vi "RT Main.vi"() -> ()   [LabVIEW 2021]
uses:
  <vilib>/FPGAPlugInAG/myRIO-1900/niLvFpga_Open_myRIO-1900.vi
  <vilib>/rvi/interface/common/dynamic/niFpgaDynamicAddResources.vi
  <vilib>/rvi/interface/common/niFpgaWaitOnOcc.vi
  <vilib>/Utility/error.llb/Error Cluster From Error Code.vi
  <vilib>/rvi/errors/niLvFpgaAdjustHostInterfaceError.vi
  <vilib>/FPGAPlugInAG/Dynamic/niLvFpga_Close_Dynamic.vi
  <vilib>/rvi/interface/nirviOpenFPGA/nirviOpenFPGA.xnode
  FPGA Bitfiles/dmafifoproject_FPGATarget_FPGA_+Bf8FZcda64.lvbitx
  <vilib>/rvi/interface/nirviMethod/nirviMethod.xnode
  <vilib>/rvi/interface/nirviReadWriteControl/nirviReadWriteControl.xnode
  <vilib>/rvi/interface/nirviCloseFPGA/nirviCloseFPGA.xnode
  <vilib>/rvi/errors/niLvFpgaMergeErrorWithErrorCode.vi
  <vilib>/FPGAPlugInAG/Dynamic/niLvFpga_ConfigureFifo_Dynamic.vi
  NiFpgaLv.dll
  <vilib>/rvi/interface/Simulation/niFpgaSimulationCallBeginRW.vi
  <vilib>/FPGAPlugInAG/Dynamic/niLvFpga_ReadFifo_Dynamic.vi
  <vilib>/FPGAPlugInAG/Dynamic/niLvFpga_WriteFifo_Dynamic.vi
panel:
  out "Waveform Chart":i16[][](graph)
  in  "min loop time [ms]":u32
  in  "stop":bool
  out "measured loop time [ms]":u32
  in  "gain":sgl
  out "to RT-Elements Remaining":u32
  in  "audio frame size [sample]":u32
  out "From RT underflow?":bool
  out "to RT overflow":bool
  out "audio sampling interval [us]":u32
  in  "audio sampling rate":dbl
  out "from RT-depth":u32
  out "to RT-depth":u32
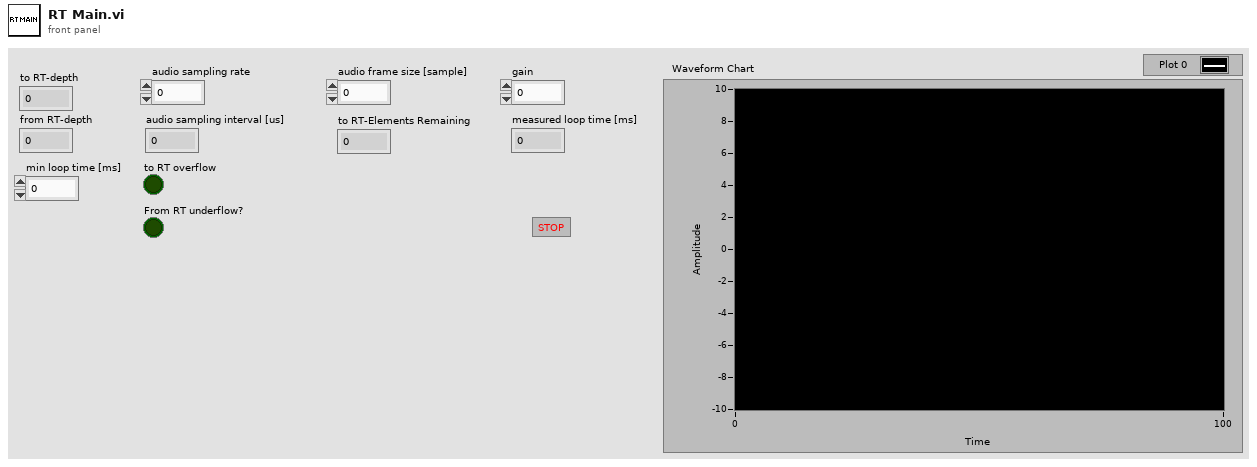
[diagram p1: front panel]
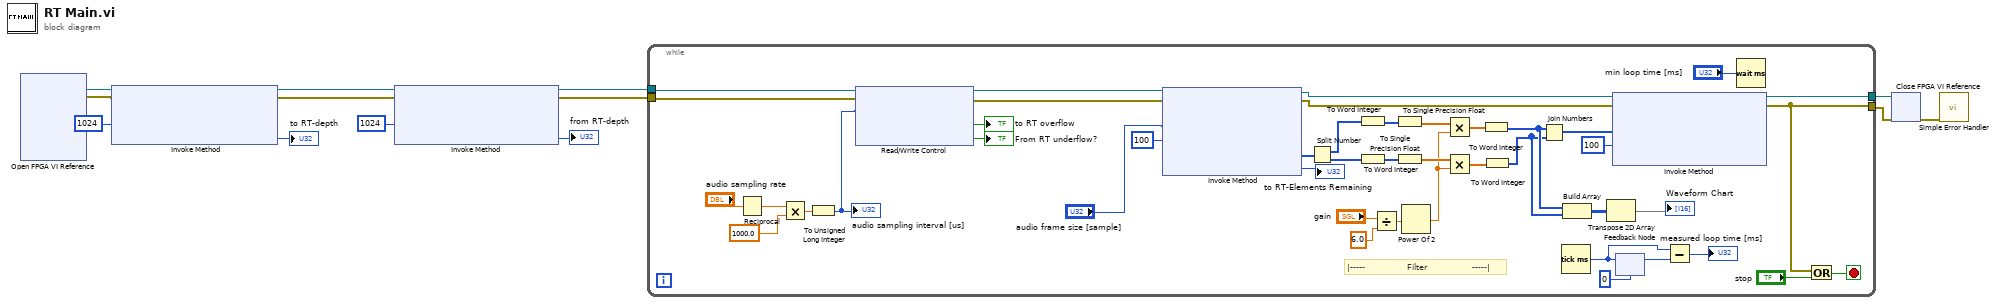
[diagram p0: block diagram]
diagram:
  n1 = xnode "Open FPGA VI Reference"() -> ("FPGA VI Reference Out"=w13:refnum<k20>, "error out"=w10:errorcluster)  [unwired: 2 in]
  n2 = xnode "Invoke Method"("FPGA VI Reference In"=w13, "error in"=w10, "Requested Depth"=u32 1024) -> ("FPGA VI Reference Out"=w12:refnum<k20>, "error out"=w11:errorcluster, "Actual Depth"=→"to RT-depth":u32)
  n3 = xnode "Invoke Method"("FPGA VI Reference In"=w12, "error in"=w11, "Requested Depth"=u32 1024) -> ("FPGA VI Reference Out"=w5:refnum<k20>, "error out"=w4:errorcluster, "Actual Depth"=→"from RT-depth":u32)
  n4 = while {
    tunnel: w5 -> [w57]
    tunnel: w4 -> [w56]
    tunnel: [w16] -> w3
    tunnel: [w17] -> w2
    stop <- w18 stop-if-true
    # "|-----              Filter               -----|"
    n5 = Reciprocal(x="audio sampling rate") -> (1/x=w52:dbl)
    n6 = Multiply(x=w52, y=1000.0) -> (x*y=w50:dbl)
    n7 = To Unsigned Long Integer(number=w50) -> (unsigned 32bit integer=w49:u32)
    "audio sampling interval [us]" <- w49
    n8 = xnode "Read/Write Control"("FPGA VI Reference In"=w57, "error in"=w56, "loop time(uSec)"=w49) -> ("FPGA VI Reference Out"=w55:refnum<k20>, "error out"=w54:errorcluster, "to RT overflow"=→"to RT overflow":bool, "From RT underflow?"=→"From RT underflow?":bool)
    n9 = xnode "Invoke Method"("FPGA VI Reference In"=w55, "error in"=w54, "Number of Elements"="audio frame size [sample]", "Timeout (ms)"=100) -> ("FPGA VI Reference Out"=w30:refnum<k20>, "error out"=w29:errorcluster, "Data"=w44:u32[], "Elements Remaining"=→"to RT-Elements Remaining":u32)
    n10 = Split Number(x=w44) -> (hi(x)=w42:u16[], lo(x)=w41:u16[])
    n11 = To Word Integer(number=w42) -> (16bit integer=w40:i16[])
    n12 = To Word Integer(number=w41) -> (16bit integer=w39:i16[])
    n13 = Divide(x="gain", y=sgl 6.0) -> (x/y=w34:sgl)
    n14 = To Single Precision Float(number=w40) -> (single precision float=w38:sgl[])
    n15 = To Single Precision Float(number=w39) -> (single precision float=w37:sgl[])
    n16 = Power Of 2(x=w34) -> (2^x=w33:sgl)
    n17 = Multiply(x=w38, y=w33) -> (x*y=w32:sgl[])
    n18 = Multiply(x=w37, y=w33) -> (x*y=w31:sgl[])
    n19 = To Word Integer(number=w32) -> (16bit integer=w26:i16[])
    n20 = To Word Integer(number=w31) -> (16bit integer=w25:i16[])
    n21 = Join Numbers(hi=w26, lo=w25) -> ((hi.lo)=w28:u32[])
    n22 = Tick Count (ms)() -> (millisecond timer value=w21:u32)
    n23 = Build Array(w26, w25) -> (w24:i16[][])
    n24 = Transpose 2D Array(2D array=w24) -> (transposed array=→"Waveform Chart":i16[][])
    n25 = xnode "Invoke Method"("FPGA VI Reference In"=w30, "error in"=w29, "Data"=w28, "Timeout (ms)"=100) -> ("FPGA VI Reference Out"=w16:refnum<k20>, "error out"=w17:errorcluster)  [unwired: 1 out]
    n26 = feedback-in #1(w21) -> ()
    n27 = feedback #1(u32 0 ("millisecond timer value")) -> (w22:u32)
    n28 = Subtract(x=w21, y=w22) -> (x-y=→"measured loop time [ms]":u32)
    n29 = Wait (ms)(milliseconds to wait="min loop time [ms]") -> ()  [unwired: 1 out]
    n30 = Or(x=w17, y="stop") -> (x .or. y?=w18:bool)
  }
  n31 = xnode "Close FPGA VI Reference"("FPGA VI Reference In"=w3, "error in"=w2) -> ("error out"=w1:errorcluster)
  n32 = call <vilib>:"Simple Error Handler.vi"("error in (no error)"=w1) -> ()  [unwired: 4 in, 5 out]
